vi "Create Sessions.vi"(8 "error in (no error)":errorcluster, 11 "Compiled Data in":T4 {"Corruption Info DUT_Network"."Frame Infos Array"."CRC Index" min=-7 max=7; "Corruption Info DUT_Network"."Frame Infos Array"."DLC Length  Corruption Index" min=-8 max=8; "Corruption Info Network_DUT"."Frame Infos Array"."CRC Index" min=-7 max=7; "Corruption Info Network_DUT"."Frame Infos Array"."DLC Length  Corruption Index" min=-8 max=8}) -> (0 "error out":errorcluster, 3 "Engine Run-Time Data Cluster":T1 {"Compiled Data"."Corruption Info DUT_Network"."Frame Infos Array"."CRC Index" min=-7 max=7; "Compiled Data"."Corruption Info DUT_Network"."Frame Infos Array"."DLC Length  Corruption Index" min=-8 max=8; "Compiled Data"."Corruption Info Network_DUT"."Frame Infos Array"."CRC Index" min=-7 max=7; "Compiled Data"."Corruption Info Network_DUT"."Frame Infos Array"."DLC Length  Corruption Index" min=-8 max=8; "Specified Channel Ref List Out" format="%.0x"; "Specified Channel Ref List In" format="%.0x"})   [LabVIEW 2018, in "CAN Gateway Engine.lvlib"]
uses:
  CAN Gateway Engine.lvlib
  Shared/CTLs/Compiled Data.ctl
  Shared/CTLs/Corruption Info.ctl
  Shared/CTLs/Frame.ctl
  Shared/CTLs/Signal_Data_Trigger.ctl
  Shared/CTLs/Runtime engine Data.ctl
  <vilib>/NI Veristand/Custom Device API/Custom Device Engine Event Ref.ctl
  <vilib>/NI Veristand/Custom Device API/Custom Device Item Ref.ctl
  <vilib>/NI Veristand/Custom Device API/Message (Byte Array).ctl
  <vilib>/NI Veristand/Custom Device API/Message Response (Byte Array).ctl
  <vilib>/NI Veristand/Custom Device API/Message (String).ctl
  <vilib>/NI Veristand/Custom Device API/Message Response (String).ctl
  <vilib>/xnet/xnet.llb/XNET Create Session (Frame Output Stream).vi
  <vilib>/xnet/xnet.llb/XNET Create Session (Frame Input Stream).vi
  <vilib>/xnet/xnet.llb/XNET Create Session (Conversion).vi
  Shared/CAN Gateway Shared.lvlib
  <vilib>/NI Veristand/Custom Device API/Custom Device API.lvlib
  <resource>/objmgr/xnet.rc
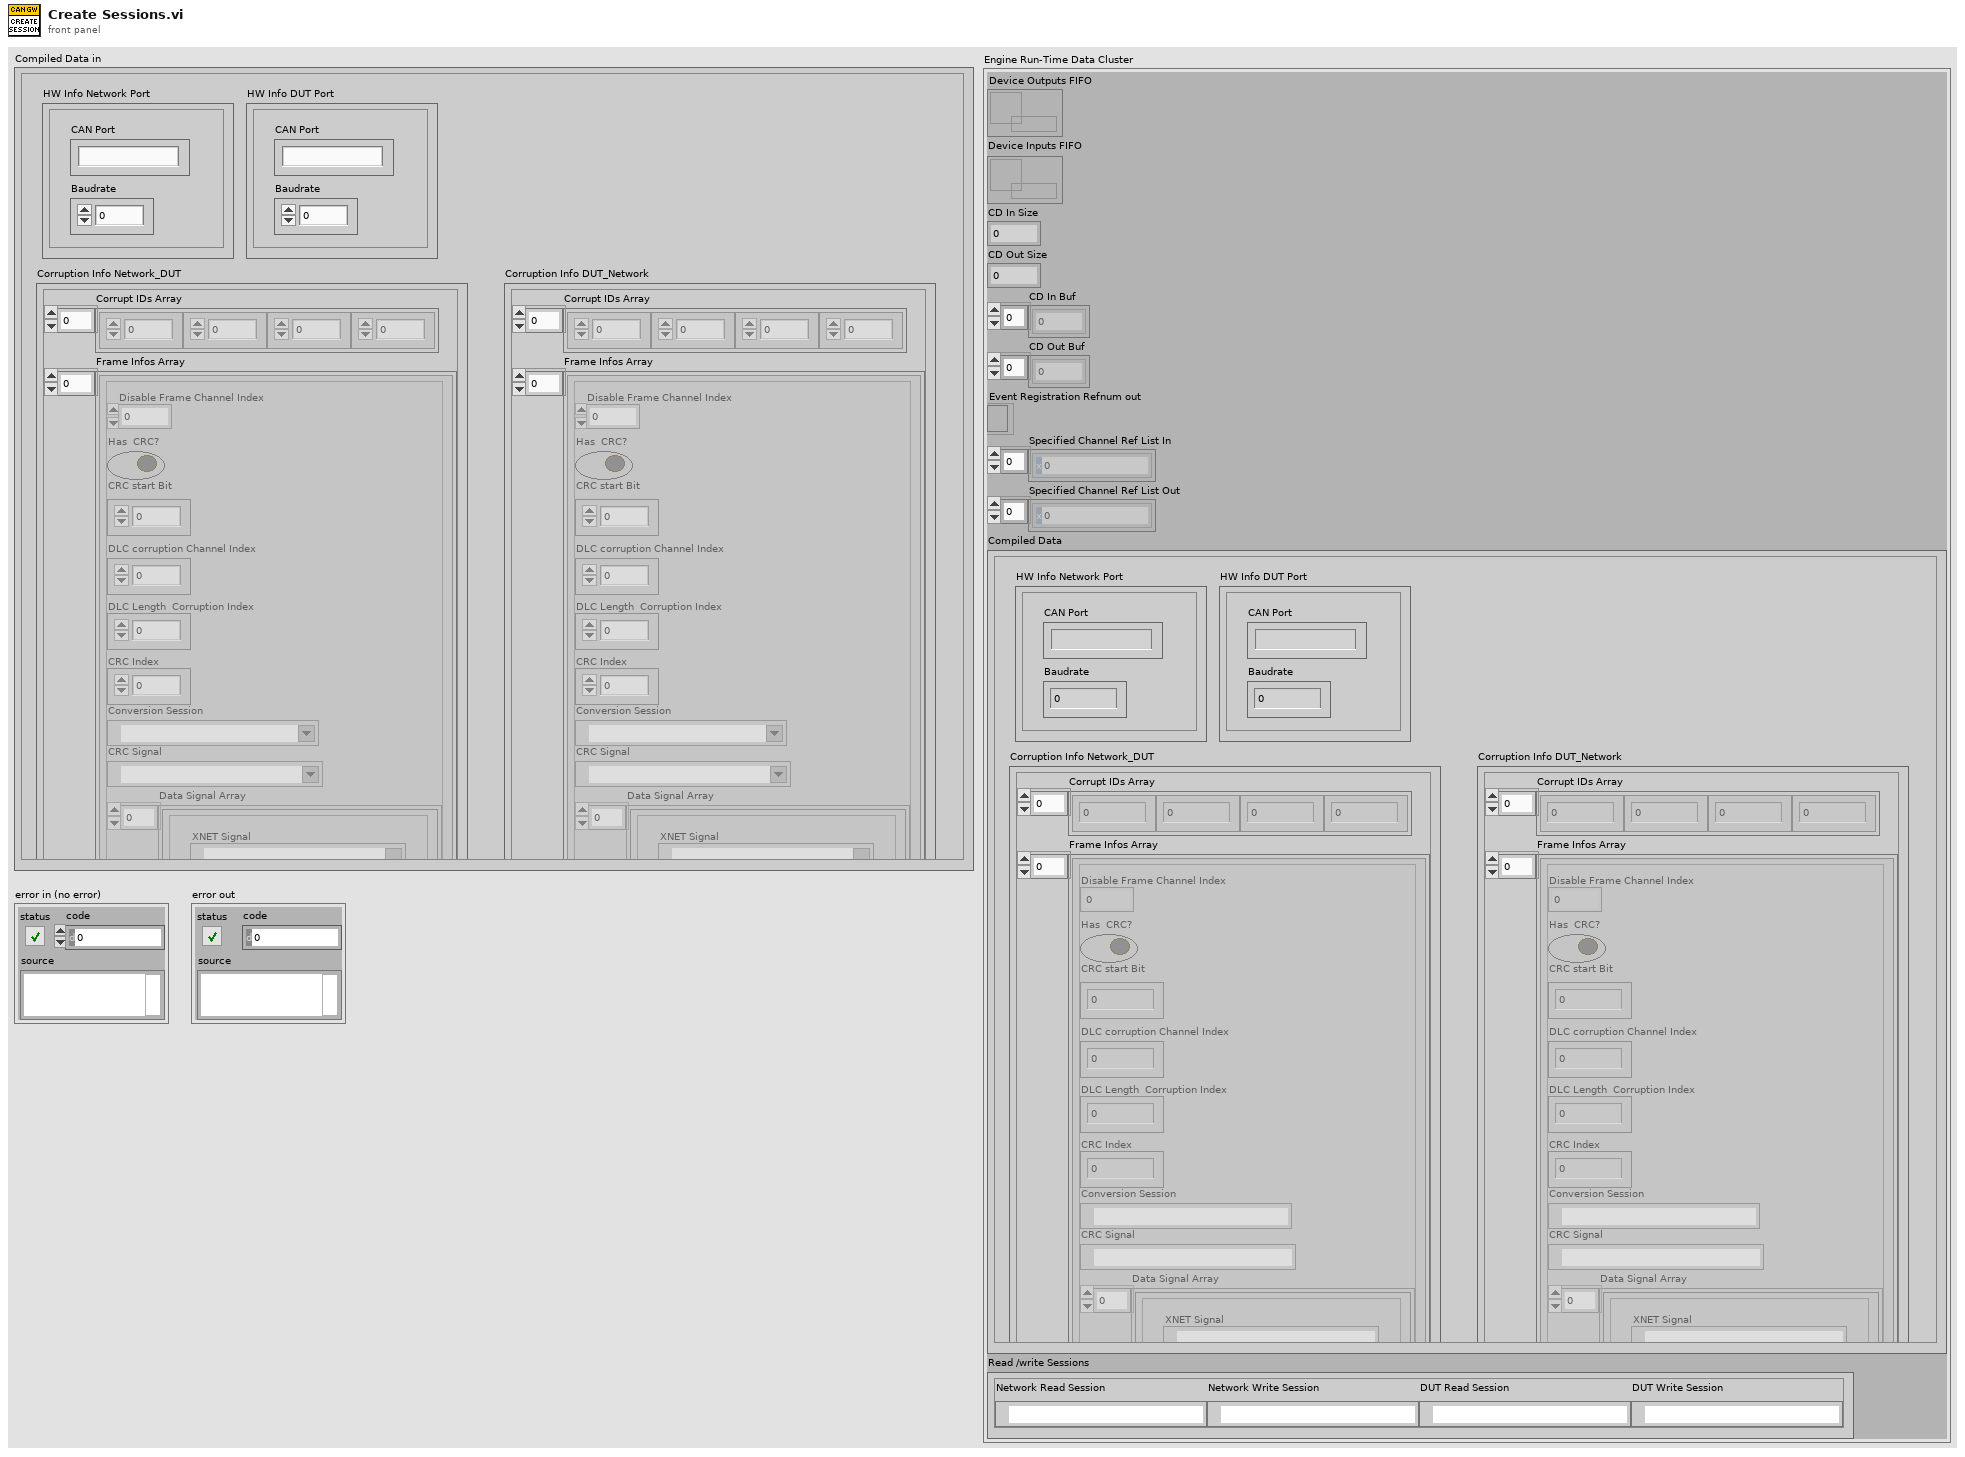
[diagram p1: front panel]
types:
  T1 = typedef "CAN Gateway Engine.lvlib/Runtime engine Data.ctl" = cluster{"Device Outputs FIFO":refnum<k33>, "Device Inputs FIFO":refnum<k33>, "CD In Size":i32, "CD Out Size":i32, "CD In Buf":dbl[], "CD Out Buf":dbl[], "Event Registration Refnum out":T2, "Specified Channel Ref List In":T3[], "Specified Channel Ref List Out":T3[], "Compiled Data":T4, "Read /write Sessions":cluster{"Network Read Session":refnum<k21>, "Network Write Session":refnum<k21>, "DUT Read Session":refnum<k21>, "DUT Write Session":refnum<k21>}}
  T2 = typedef "Custom Device API.lvlib/Custom Device Engine Event Ref.ctl" = refnum<event-registration>
  T3 = typedef "Custom Device API.lvlib/Custom Device Item Ref.ctl" = u64
  T4 = typedef "CAN Gateway Shared.lvlib/Compiled Data.ctl" = cluster{"HW Info Network Port":cluster{"CAN Port":string, "Baudrate":u64}, "HW Info DUT Port":cluster{"CAN Port":string, "Baudrate":u64}, "Corruption Info Network_DUT":T5, "Corruption Info DUT_Network":T5}
  T5 = typedef "CAN Gateway Shared.lvlib/Corruption Info.ctl" = cluster{"Corrupt IDs Array":u32[], "Frame Infos Array":T6[]}
  T6 = typedef "CAN Gateway Shared.lvlib/Frame.ctl" = cluster{"Disable Frame Channel Index":i32, "Has  CRC?":bool, "CRC start Bit":u32, "DLC corruption Channel Index":i32, "DLC Length  Corruption Index":i32, "CRC Index":i32, "Conversion Session":refnum<k21>, "CRC Signal":refnum<k21>, "Data Signal Array":T7[]}
  T7 = typedef "CAN Gateway Shared.lvlib/Signal_Data_Trigger.ctl" = cluster{"XNET Signal":refnum<k21>, "Data Idx":u32, "Trigger Idx":u32}
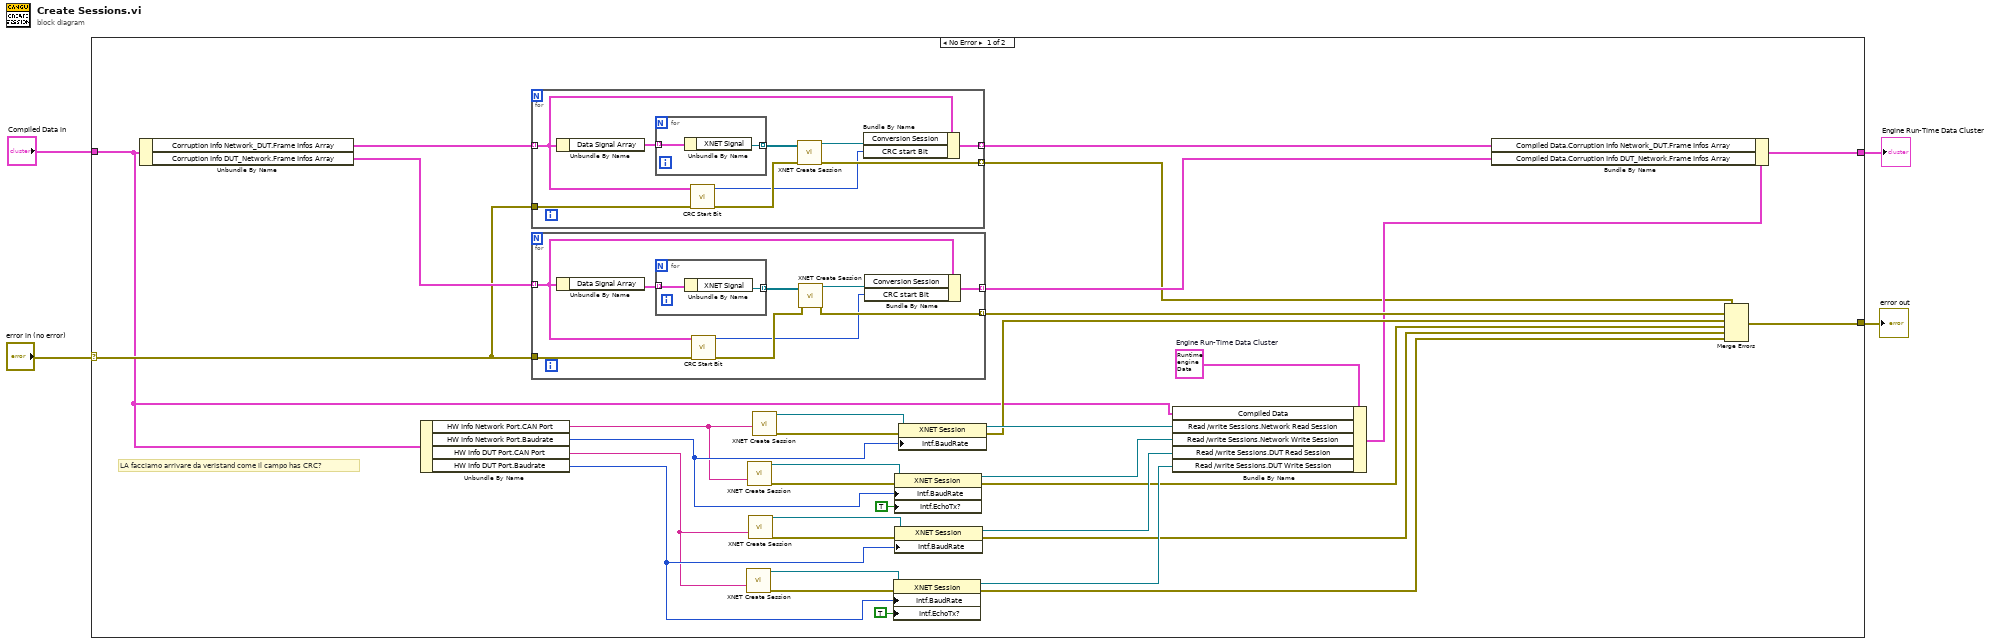
[diagram p0: block diagram]
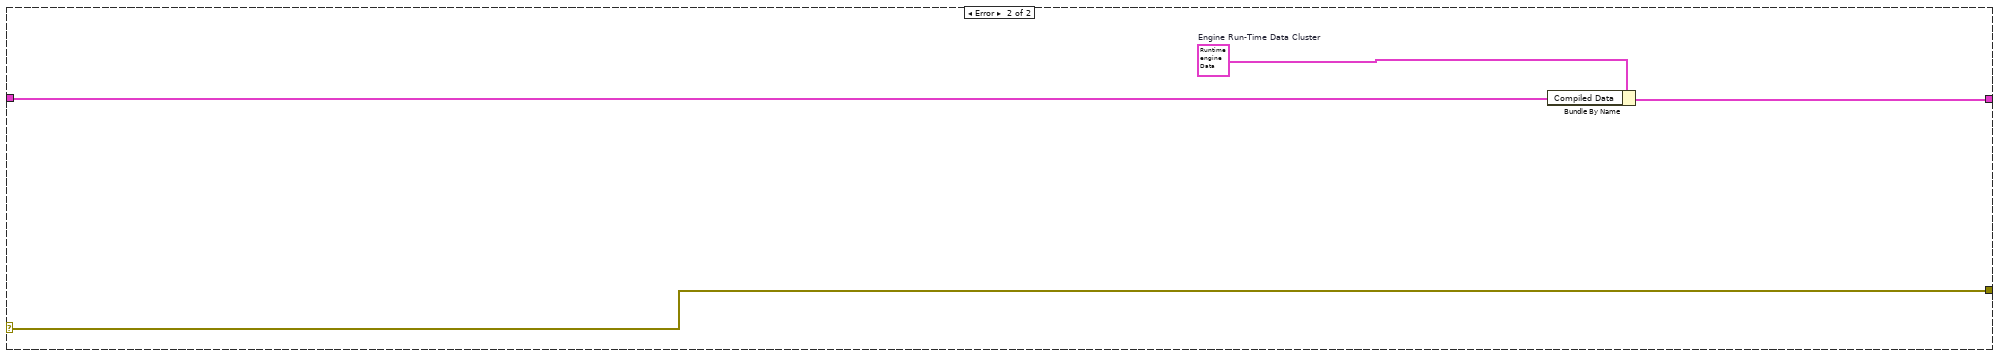
[diagram p2: hidden frame]
diagram:
  n1 = case shown="No Error" "error in (no error)" {
    selector: "error in (no error)" -> [w12 w64]
    tunnel: [w24 w62] -> w1
    tunnel: "Compiled Data in" -> [w7 w61]
    tunnel: [w36 w64] -> w3
    frame No Error {
      w15 = T1 {"Device Outputs FIFO"=refnum, "Device Inputs FIFO"=refnum, "CD In Size"=0, "CD Out Size"=0, "CD In Buf"=[], "CD Out Buf"=[], "Event Registration Refnum out"=refnum, "Specified Channel Ref List In"=[], "Specified Channel Ref List Out"=[], "Compiled Data"={"HW Info Network Port"={"CAN Port"="", "Baudrate"=0}, "HW Info DUT Port"={"CAN Port"="", "Baudrate"=0}, "Corruption Info Network_DUT"={"Corrupt IDs Array"=[], "Frame Infos Array"=[]}, "Corruption Info DUT_Network"={"Corrupt IDs Array"=[], "Frame Infos Array"=[]}}, "Read /write Sessions"={"Network Read Session"="", "Network Write Session"="", "DUT Read Session"="", "DUT Write Session"=""}}  # Engine Run-Time Data Cluster
      # "LA facciamo arrivare da veristand come il campo has CRC?"
      n2 = Unbundle By Name(w7) -> ("Corruption Info Network_DUT.Frame Infos Array"=w13:T6[], "Corruption Info DUT_Network.Frame Infos Array"=w38:T6[])
      n3 = Unbundle By Name(w7) -> ("HW Info Network Port.CAN Port"=w8:string, "HW Info Network Port.Baudrate"=w27:u64, "HW Info DUT Port.CAN Port"=w9:string, "HW Info DUT Port.Baudrate"=w26:u64)
      n4 = for {
        tunnel: w13 -> [w39] mode=indexing
        tunnel: [w44] -> w11 mode=indexing
        tunnel: w12 -> [w40]
        tunnel: [w43] -> w10 mode=indexing
        n5 = Unbundle By Name(w39) -> ("Data Signal Array"=w47:T7[])
        n6 = for {
          tunnel: w47 -> [w49] mode=indexing
          tunnel: [w48] -> w46 mode=indexing
          n7 = Unbundle By Name(w49) -> ("XNET Signal"=w48:refnum<k21>)
        }
        n8 = call "CRC Start Bit.vi"("error in (no error)"=w40, "Frame Infos"=w39) -> ("error out"=w42:errorcluster, "CRC Start Bit"=w41:u32)  [unwired: 8 in]
        n9 = call-poly <vilib>:"XNET Create Session.vi"("signal list"=w46, "error in (no error)"=w42) -> ("session out"=w45:refnum<k21>, "error out"=w43:errorcluster)  [unwired: 12 in]
        n10 = Bundle By Name(cluster=w39, "Conversion Session"=w45, "CRC start Bit"=w41) -> (w44:T6)
      }
      n11 = for {
        tunnel: w38 -> [w50] mode=indexing
        tunnel: [w55] -> w25 mode=indexing
        tunnel: w12 -> [w51]
        tunnel: [w54] -> w37 mode=indexing
        n12 = Unbundle By Name(w50) -> ("Data Signal Array"=w58:T7[])
        n13 = for {
          tunnel: w58 -> [w60] mode=indexing
          tunnel: [w59] -> w57 mode=indexing
          n14 = Unbundle By Name(w60) -> ("XNET Signal"=w59:refnum<k21>)
        }
        n15 = call "CRC Start Bit.vi"("error in (no error)"=w51, "Frame Infos"=w50) -> ("error out"=w53:errorcluster, "CRC Start Bit"=w52:u32)  [unwired: 8 in]
        n16 = call-poly <vilib>:"XNET Create Session.vi"("signal list"=w57, "error in (no error)"=w53) -> ("session out"=w56:refnum<k21>, "error out"=w54:errorcluster)  [unwired: 12 in]
        n17 = Bundle By Name(cluster=w50, "Conversion Session"=w56, "CRC start Bit"=w52) -> (w55:T6)
      }
      n18 = call-poly <vilib>:"XNET Create Session.vi"("interface"=w9) -> ("session out"=w28:refnum<k21>, "error out"=w29:errorcluster)  [unwired: 13 in]
      n19 = call-poly <vilib>:"XNET Create Session.vi"("interface"=w8) -> ("session out"=w32:refnum<k21>, "error out"=w33:errorcluster)  [unwired: 13 in]
      n20 = call-poly <vilib>:"XNET Create Session.vi"("interface"=w9) -> ("session out"=w31:refnum<k21>, "error out"=w30:errorcluster)  [unwired: 13 in]
      n21 = call-poly <vilib>:"XNET Create Session.vi"("interface"=w8) -> ("session out"=w35:refnum<k21>, "error out"=w34:errorcluster)  [unwired: 13 in]
      n22 = property class="XNET Session"(reference=w28, error in=w29, "Intf.BaudRate"=w26, "Intf.EchoTx?"=TRUE ("Interface:Echo Transmit?")) -> (reference out=w20:refnum<k21>, error out=w16:errorcluster)
      n23 = property class="XNET Session"(reference=w32, error in=w33, "Intf.BaudRate"=w27, "Intf.EchoTx?"=TRUE ("Interface:Echo Transmit?")) -> (reference out=w22:refnum<k21>, error out=w18:errorcluster)
      n24 = property class="XNET Session"(reference=w31, error in=w30, "Intf.BaudRate"=w26) -> (reference out=w21:refnum<k21>, error out=w17:errorcluster)
      n25 = property class="XNET Session"(reference=w35, error in=w34, "Intf.BaudRate"=w27) -> (reference out=w23:refnum<k21>, error out=w19:errorcluster)
      n26 = Bundle By Name(cluster=w15, "Compiled Data"=w7, "Read /write Sessions.Network Read Session"=w23, "Read /write Sessions.Network Write Session"=w22, "Read /write Sessions.DUT Read Session"=w21, "Read /write Sessions.DUT Write Session"=w20) -> (w14:T1)
      n27 = Bundle By Name(cluster=w14, "Compiled Data.Corruption Info Network_DUT.Frame Infos Array"=w11, "Compiled Data.Corruption Info DUT_Network.Frame Infos Array"=w25) -> (w24:T1)
      n28 = Merge Errors(w10, w37, w19, w18, w17, w16) -> (w36:errorcluster)
    }
    frame Error {
      w63 = T1 {"Device Outputs FIFO"=refnum, "Device Inputs FIFO"=refnum, "CD In Size"=0, "CD Out Size"=0, "CD In Buf"=[], "CD Out Buf"=[], "Event Registration Refnum out"=refnum, "Specified Channel Ref List In"=[], "Specified Channel Ref List Out"=[], "Compiled Data"={"HW Info Network Port"={"CAN Port"="", "Baudrate"=0}, "HW Info DUT Port"={"CAN Port"="", "Baudrate"=0}, "Corruption Info Network_DUT"={"Corrupt IDs Array"=[], "Frame Infos Array"=[]}, "Corruption Info DUT_Network"={"Corrupt IDs Array"=[], "Frame Infos Array"=[]}}, "Read /write Sessions"={"Network Read Session"="", "Network Write Session"="", "DUT Read Session"="", "DUT Write Session"=""}}  # Engine Run-Time Data Cluster
      n29 = Bundle By Name(cluster=w63, "Compiled Data"=w61) -> (w62:T1)
    }
  }
  "error out" <- w3
  "Engine Run-Time Data Cluster" <- w1
